vi "RPMtoSpeed.vi"(10 "RPM":dbl) -> (2 "Speed":dbl)   [LabVIEW 2012]
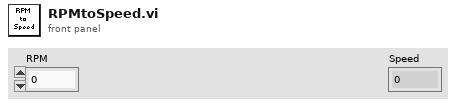
[diagram p1: front panel]
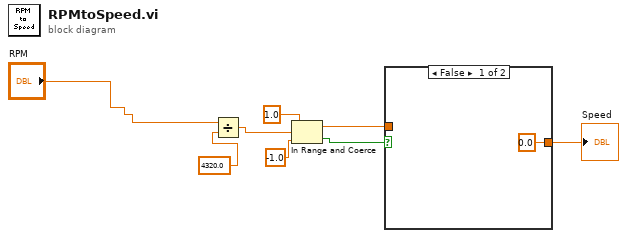
[diagram p0: block diagram]
diagram:
  n1 = Divide(x="RPM", y=4320.0) -> (x/y=w5:dbl)
  n2 = In Range and Coerce(upper limit=1.0, x=w5, lower limit=-1.0) -> (coerced(x)=w3:dbl, In Range?=w4:bool)
  n3 = case shown="False" w4 {
    tunnel: w3 -> [_ w10]
    tunnel: [0.0 ("upper limit") w10] -> w1
    frame False {
    }
    frame True {
    }
  }
  "Speed" <- w1
